vi "parser error.vi"(0 "string in":string) -> (1 "Boolean":bool)   [LabVIEW 2013]
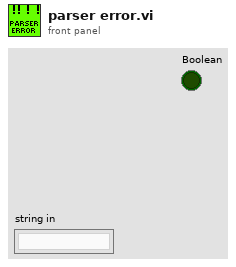
[diagram p1: front panel]
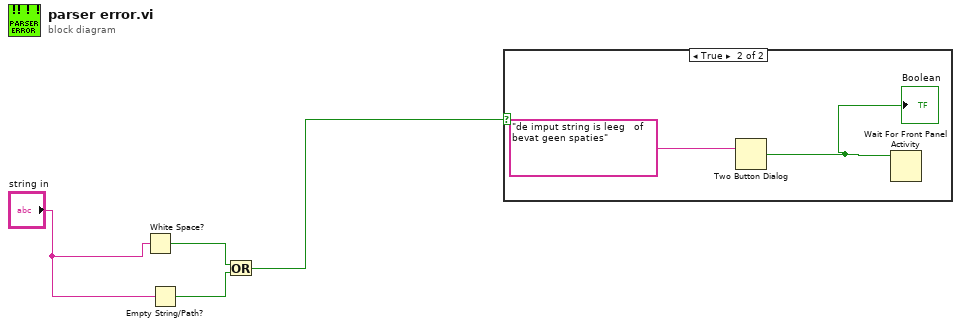
[diagram p0: block diagram]
diagram:
  n1 = White Space?(1:"string in") -> (0:w1:bool)
  n2 = Empty String/Path?(string/path="string in") -> (empty?=w4:bool)
  n3 = Or(x=w1, y=w4) -> (x .or. y?=w2:bool)
  n4 = case shown="True" w2 {
    frame False {
    }
    frame True {
      n5 = Two Button Dialog(message="de imput string is leeg   of bevat geen spaties") -> (T button?=w5:bool)  [unwired: 2 in]
      "Boolean" <- w5
      n6 = Wait For Front Panel Activity(3:w5) -> ()  [unwired: 2 in, 1 out]
    }
  }
